vi "MKS670_100_Main.vi"(7 "stop_external":refnum<vi>, 8 "input cluster":T1) -> ()   [LabVIEW 2019]
uses:
  cluster_ref_MKS670.ctl
panel:
  out "P Chart":waveform(dbl)[](graph)
  in  "Meas. Interval":u32=1000 caption="ms"
  out "Status":bool
  out "Last Updated":timestamp format="%<%Y-%m-%d %H:%M:%S>T"
  out "Version":dbl
  out "Pressure":dbl caption="Torr"
  out "Name":string
  in  "stop":bool
  out "Message":string
  in  "GPIB":string="1:7"
  # "MKS 670 for MKS 690 / 100 Torr"
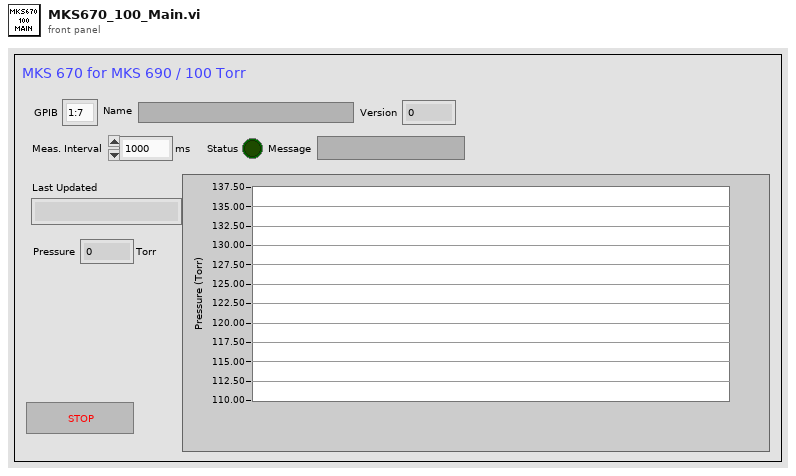
[diagram p1: front panel]
types:
  T1 = typedef "cluster_ref_MKS670.ctl" = cluster{"status":refnum<vi>, "PR":refnum<vi>}
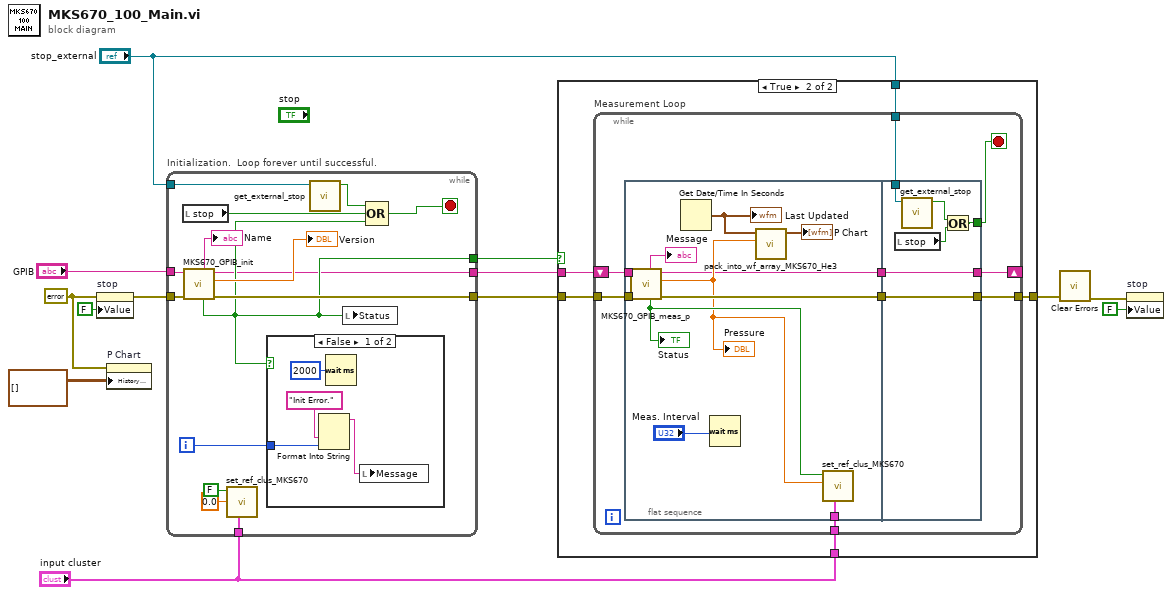
[diagram p0: block diagram]
diagram:
  w3 = errorcluster {"status"=FALSE, "code"=0, "source"=""} ("error in")
  n1 = property on="stop" class="Bool (strict)"(error in=w3, "Value"=FALSE ("stop")) -> (error out=w11:errorcluster)  [unwired: 1 in, 1 out]
  n2 = property on="P Chart" class="WFChart (strict)"(error in=w3, "History Data"=waveform(dbl)[][] []) -> ()  [unwired: 1 in, 2 out]
  n3 = while "Initialization.  Loop forever until successful." {
    tunnel: w11 -> [w27]
    tunnel: "GPIB" -> [w26]
    tunnel: [w25] -> w9
    tunnel: "stop_external" -> [w20]
    tunnel: [w18] -> w8
    tunnel: "input cluster" -> [w17]
    tunnel: [w14] -> w1
    i -> [w23]
    stop <- w22 stop-if-true
    n4 = local read "stop"() -> (w21:bool)
    n5 = call "MKS670_GPIB_init.vi"("error in (no error)"=w27, "GPIB Address"=w26) -> ("error out"=w25:errorcluster, "Device Version"=→"Version":dbl, "GPIB out"=w14:string, "status"=w18:bool, "Device Name"=→"Name":string)  [unwired: 5 in]
    n6 = call "set_ref_clus_MKS670.vi"("input cluster"=w17, "pressure"=0.0, "status"=FALSE) -> ()  [unwired: 9 in]
    n7 = case shown="False" w18 {
      tunnel: w23 -> [w30 _]
      frame False {
        n8 = Format Into String("Init Error.", w30) -> (resulting string=w31:string)  [unwired: 3 in, 1 out]
        n9 = Wait (ms)(milliseconds to wait=u32 2000) -> ()  [unwired: 1 out]
        n10 = local write "Message"(w31) -> ()
      }
      frame True {
      }
    }
    n11 = call "get_external_stop.vi"("ref_stop_external"=w20) -> ("stop_output"=w19:bool)  [unwired: 10 in]
    n12 = local write "Status"(w18) -> ()
    n13 = Compound Arithmetic op=OR(w19, w21, w18) -> (w22:bool)
  }
  n14 = case shown="True" w8 {
    tunnel: "stop_external" -> [_ w38]
    tunnel: w9 -> [w33 w37]
    tunnel: [w33 w36] -> w6
    tunnel: "input cluster" -> [_ w35]
    tunnel: w1 -> [_ w34]
    frame False {
    }
    frame True {
      n15 = while "Measurement Loop" {
        tunnel: w37 -> [w47]
        tunnel: w38 -> [w40]
        tunnel: [w46] -> w36
        tunnel: w35 -> [w45]
        shift-right: [w43] -> _
        shift-left: w34 -> [w44]
        stop <- w39 stop-if-true
        n16 = flat-sequence {
          tunnel: w47 -> [w58]
          tunnel: w45 -> [w54]
          tunnel: w44 -> [w49]
          tunnel: [w55] -> w42
          tunnel: [w48] -> w41
          tunnel: [w63] -> w43
          tunnel: [w64] -> w46
          tunnel: w42 -> [w64]
          tunnel: w41 -> [w63]
          tunnel: w40 -> [w60]
          tunnel: [w59] -> w39
          frame #0 {
            n17 = call "MKS670_GPIB_meas_p.vi"("error in"=w58, "GPIB Address"=w49) -> ("error out"=w55:errorcluster, "value"=w52:dbl, "GPIB out"=w48:string, "status"=w53:bool, "msg"=→"Message":string)  [unwired: 5 in]
            "Status" <- w53
            "Pressure" <- w52
            n18 = Get Date/Time In Seconds() -> (seconds since 1Jan1904=w57:timestamp)
            "Last Updated" <- w57
            n19 = Wait (ms)(milliseconds to wait="Meas. Interval") -> ()  [unwired: 1 out]
            n20 = call "pack_into_wf_array_MKS670_He3.vi"("pressure"=w52, "time"=w57) -> ("waveform_array"=→"P Chart":waveform(dbl)[])  [unwired: 9 in]
            n21 = call "set_ref_clus_MKS670.vi"("input cluster"=w54, "pressure"=w52, "status"=w53) -> ()  [unwired: 9 in]
          }
          frame #1 {
            n22 = local read "stop"() -> (w62:bool)
            n23 = call "get_external_stop.vi"("ref_stop_external"=w60) -> ("stop_output"=w61:bool)  [unwired: 10 in]
            n24 = Or(x=w61, y=w62) -> (x .or. y?=w59:bool)
          }
        }
      }
    }
  }
  n25 = call <vilib>:"Clear Errors.vi"("error in (no error)"=w6) -> ("error out"=w5:errorcluster)  [unwired: 5 in, 1 out]
  n26 = property on="stop" class="Bool (strict)"(error in=w5, "Value"=FALSE ("stop")) -> ()  [unwired: 1 in, 2 out]
